vi "Write TestLog.vi"(10 "ITestLog.lvclass":refnum<class "ITestLog.lvclass">, 11 "Model in":refnum<class "Model.lvclass">) -> (3 "Model out":refnum<class "Model.lvclass">)   [LabVIEW 2015, in "Model.lvclass"]
uses:
  Model.lvclass
  TestLog/ITestLog/ITestLog.lvclass
  Model.lvclass/Model.ctl
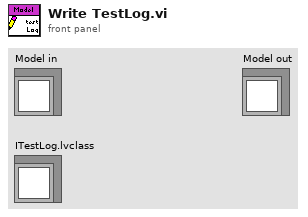
[diagram p1: front panel]
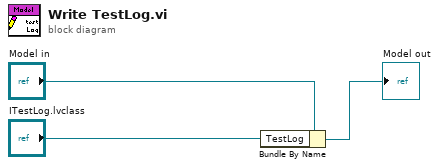
[diagram p0: block diagram]
diagram:
  n1 = Bundle By Name(cluster="Model in", "TestLog"="ITestLog.lvclass") -> (→"Model out":refnum<class "Model.lvclass">)
